vi "КАЛЬКУЛЯТОР.vi"() -> ()   [LabVIEW 2012]
uses:
  Control 1.ctl
panel:
  out "Boolean":bool
  in  ",":bool
  in  "+/-":bool
  in  "1/x":bool
  in  "CE":bool
  in  "C":bool
  in  "Backspace":bool
  in  "MS":bool
  in  "MR":bool
  in  "MC":bool
  in  "x^2":bool
  in  "sqrt":bool
  in  "/":bool
  in  "*":bool
  in  "-":bool
  in  "0":bool
  in  "9":bool
  in  "8":bool
  in  "7":bool
  in  "6":bool
  in  "5":bool
  in  "4":bool
  in  "3":bool
  out "екран":string
  in  "=":bool
  in  "+":bool
  in  "2":bool
  in  "1":bool
  in  "stop":bool
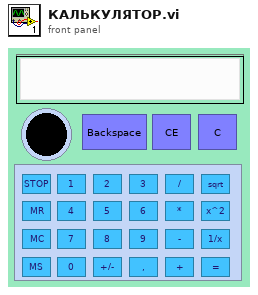
[diagram p1: front panel]
types:
  T1 = typedef "Control 1.ctl" = enum16{",", "+/-", "1/x", "Backspace", "CE", "C", "MC", "MR", "MS", "x^2", "sqrt", "поділити", "помножити", "відняти", "0", "9", "8", "7", "6", "5", "4", "3", "1", "2", "додати", "дорівнює", "стоп"}
  T2 = cluster{"екран":string, "чис ек":string, "буф":string, "Enum":T1, "MR":string, "MS":string}
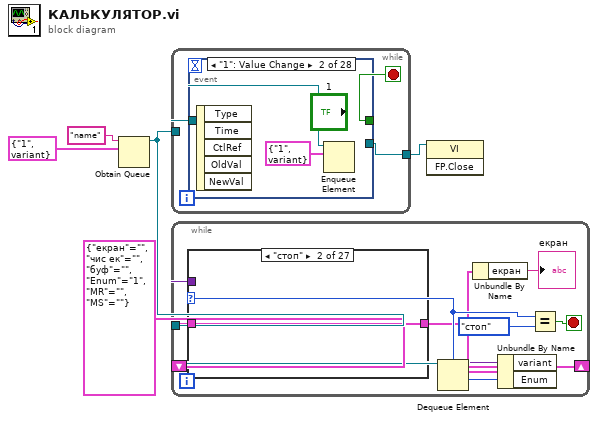
[diagram p0: block diagram]
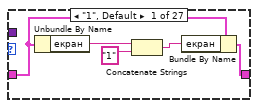
[diagram p2: hidden frame]
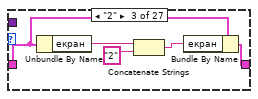
[diagram p3: hidden frame]
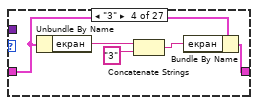
[diagram p4: hidden frame]
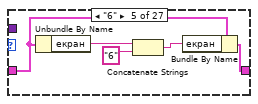
[diagram p5: hidden frame]
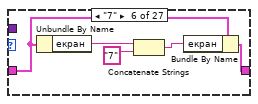
[diagram p6: hidden frame]
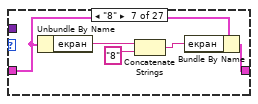
[diagram p7: hidden frame]
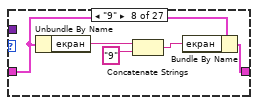
[diagram p8: hidden frame]
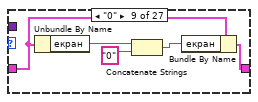
[diagram p9: hidden frame]
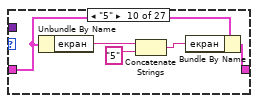
[diagram p10: hidden frame]
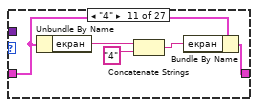
[diagram p11: hidden frame]
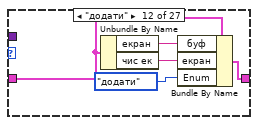
[diagram p12: hidden frame]
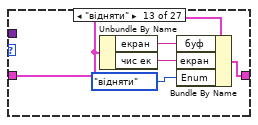
[diagram p13: hidden frame]
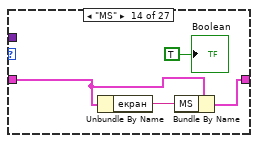
[diagram p14: hidden frame]
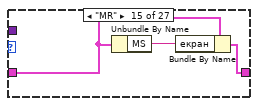
[diagram p15: hidden frame]
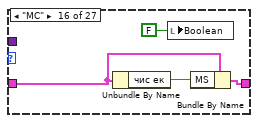
[diagram p16: hidden frame]
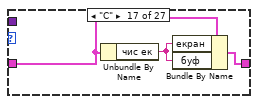
[diagram p17: hidden frame]
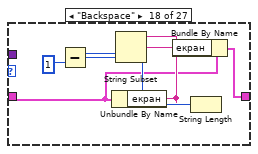
[diagram p18: hidden frame]
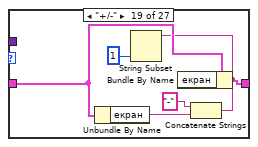
[diagram p19: hidden frame]
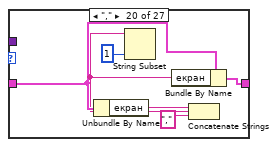
[diagram p20: hidden frame]
diagram:
  n1 = Obtain Queue(name (unnamed)="name", element data type=cluster{"Enum":T1, "variant":variant} {"Enum"=enum."1", "variant"=variant}) -> (queue out=w3:refnum<queue>)  [unwired: 3 in, 2 out]
  n2 = while {
    tunnel: w3 -> [w8]
    tunnel: [w6] -> w1
    stop <- w7 stop-if-true
    n3 = event shown="[1] \"1\": Value Change" {
      selector: _ -> [_ _ _ _ _ _ _ _ _ _ _ _ _ _ _ _ _ _ _ _ _ _ _ _ _ _ _ _]
      dyn-events: _ -> [_ _ _ _ _ _ _ _ _ _ _ _ _ _ _ _ _ _ _ _ _ _ _ _ _ _ _ _]
      timeout: _ -> [_ _ _ _ _ _ _ _ _ _ _ _ _ _ _ _ _ _ _ _ _ _ _ _ _ _ _ _]
      tunnel: w8 -> [w11 w14 w15 w17 w19 w21 w23 w25 w29 w43 w45 w47 w49 w52 w54 w56 w58 w60 w62 w64 w66 w68 w70 w72 w74 w76 w77 w80]
      tunnel: ["stop" _ _ _ _ _ _ _ w27 _ _ _ _ _ _ _ _ _ _ _ _ _ _ _ _ _ _ _] -> w7
      tunnel: [w10 _ _ _ _ _ _ _ w28 _ _ _ _ _ _ _ _ _ _ _ _ _ _ _ _ _ _ _] -> w6
      event "stop": Value Change {
        n4 = event-data() -> ()  [unwired: 1 in, 2 out]
        n5 = Enqueue Element(queue=w11, element=cluster{"Enum":T1, "variant":variant} {"Enum"=enum."стоп", "variant"=variant}) -> ()  [unwired: 2 in, 3 out]
        n6 = control-ref of="This VI"() -> (w10:refnum<vi>)
      }
      event "1": Value Change {
        n7 = event-data() -> ()  [unwired: 1 in, 5 out]
        n8 = Enqueue Element(queue=w14, element=cluster{"Enum":T1, "variant":variant} {"Enum"=enum."1", "variant"=variant}) -> ()  [unwired: 2 in, 3 out]
      }
      event "3": Value Change {
        n9 = event-data() -> ()  [unwired: 1 in, 5 out]
        n10 = Enqueue Element(queue=w15, element=cluster{"Enum":T1, "variant":variant} {"Enum"=enum."3", "variant"=variant}) -> ()  [unwired: 2 in, 3 out]
      }
      event "4": Value Change {
        n11 = event-data() -> ()  [unwired: 1 in, 5 out]
        n12 = Enqueue Element(queue=w17, element=cluster{"Enum":T1, "variant":variant} {"Enum"=enum."4", "variant"=variant}) -> ()  [unwired: 2 in, 3 out]
      }
      event "+/-": Value Change {
        n13 = event-data() -> ()  [unwired: 1 in, 5 out]
        n14 = Enqueue Element(queue=w19, element=cluster{"Enum":T1, "variant":variant} {"Enum"=enum."+/-", "variant"=variant}) -> ()  [unwired: 2 in, 3 out]
      }
      event ",": Value Change {
        n15 = event-data() -> ()  [unwired: 1 in, 5 out]
        n16 = Enqueue Element(queue=w21, element=cluster{"Enum":T1, "variant":variant} {"Enum"=enum.",", "variant"=variant}) -> ()  [unwired: 2 in, 3 out]
      }
      event "5": Value Change {
        n17 = event-data() -> ()  [unwired: 1 in, 5 out]
        n18 = Enqueue Element(queue=w23, element=cluster{"Enum":T1, "variant":variant} {"Enum"=enum."5", "variant"=variant}) -> ()  [unwired: 2 in, 3 out]
      }
      event "0": Value Change {
        n19 = event-data() -> ()  [unwired: 1 in, 5 out]
        n20 = Enqueue Element(queue=w25, element=cluster{"Enum":T1, "variant":variant} {"Enum"=enum."0", "variant"=variant}) -> ()  [unwired: 2 in, 3 out]
      }
      event Menu Selection (User) {
        n21 = event-data() -> ("ItemTag"=w30:string)  [unwired: 1 in, 5 out]
        n22 = case shown="\"False\", Default" w30 {
          tunnel: w29 -> [_ w31 w33 w35 w37 w41]
          tunnel: [_ _ _ _ _ w40] -> w28
          tunnel: [_ _ _ _ _ TRUE] -> w27
          frame "False", Default {
          }
          frame "відняти" {
            n23 = Enqueue Element(queue=w31, element=cluster{"Enum":T1, "variant":variant} {"Enum"=enum."відняти", "variant"=variant}) -> ()  [unwired: 2 in, 3 out]
          }
          frame "додати" {
            n24 = Enqueue Element(queue=w33, element=cluster{"Enum":T1, "variant":variant} {"Enum"=enum."додати", "variant"=variant}) -> ()  [unwired: 2 in, 3 out]
          }
          frame "помножити" {
            n25 = Enqueue Element(queue=w35, element=cluster{"Enum":T1, "variant":variant} {"Enum"=enum."помножити", "variant"=variant}) -> ()  [unwired: 2 in, 3 out]
          }
          frame "поділити" {
            n26 = Enqueue Element(queue=w37, element=cluster{"Enum":T1, "variant":variant} {"Enum"=enum."поділити", "variant"=variant}) -> ()  [unwired: 2 in, 3 out]
          }
          frame "стоп" {
            n27 = control-ref of="This VI"() -> (w40:refnum<vi>)
            n28 = Enqueue Element(queue=w41, element=cluster{"Enum":T1, "variant":variant} {"Enum"=enum."стоп", "variant"=variant}) -> ()  [unwired: 2 in, 3 out]
          }
        }
      }
      event "6": Value Change {
        n29 = event-data() -> ()  [unwired: 1 in, 5 out]
        n30 = Enqueue Element(queue=w43, element=cluster{"Enum":T1, "variant":variant} {"Enum"=enum."6", "variant"=variant}) -> ()  [unwired: 2 in, 3 out]
      }
      event "7": Value Change {
        n31 = event-data() -> ()  [unwired: 1 in, 5 out]
        n32 = Enqueue Element(queue=w45, element=cluster{"Enum":T1, "variant":variant} {"Enum"=enum."7", "variant"=variant}) -> ()  [unwired: 2 in, 3 out]
      }
      event "8": Value Change {
        n33 = event-data() -> ()  [unwired: 1 in, 5 out]
        n34 = Enqueue Element(queue=w47, element=cluster{"Enum":T1, "variant":variant} {"Enum"=enum."8", "variant"=variant}) -> ()  [unwired: 2 in, 3 out]
      }
      event "9": Value Change {
        n35 = event-data() -> ()  [unwired: 1 in, 5 out]
        n36 = Enqueue Element(queue=w49, element=cluster{"Enum":T1, "variant":variant} {"Enum"=enum."9", "variant"=variant}) -> ()  [unwired: 2 in, 3 out]
      }
      event "+": Value Change {
        n37 = event-data() -> ()  [unwired: 1 in, 5 out]
        n38 = Enqueue Element(queue=w52, element=cluster{"Enum":T1, "variant":variant} {"Enum"=enum."додати", "variant"=variant}) -> ()  [unwired: 2 in, 3 out]
      }
      event "-": Value Change {
        n39 = event-data() -> ()  [unwired: 1 in, 5 out]
        n40 = Enqueue Element(queue=w54, element=cluster{"Enum":T1, "variant":variant} {"Enum"=enum."відняти", "variant"=variant}) -> ()  [unwired: 2 in, 3 out]
      }
      event "*": Value Change {
        n41 = event-data() -> ()  [unwired: 1 in, 5 out]
        n42 = Enqueue Element(queue=w56, element=cluster{"Enum":T1, "variant":variant} {"Enum"=enum."помножити", "variant"=variant}) -> ()  [unwired: 2 in, 3 out]
      }
      event "/": Value Change {
        n43 = event-data() -> ()  [unwired: 1 in, 5 out]
        n44 = Enqueue Element(queue=w58, element=cluster{"Enum":T1, "variant":variant} {"Enum"=enum."поділити", "variant"=variant}) -> ()  [unwired: 2 in, 3 out]
      }
      event "sqrt": Value Change {
        n45 = event-data() -> ()  [unwired: 1 in, 5 out]
        n46 = Enqueue Element(queue=w60, element=cluster{"Enum":T1, "variant":variant} {"Enum"=enum."sqrt", "variant"=variant}) -> ()  [unwired: 2 in, 3 out]
      }
      event "x^2": Value Change {
        n47 = event-data() -> ()  [unwired: 1 in, 5 out]
        n48 = Enqueue Element(queue=w62, element=cluster{"Enum":T1, "variant":variant} {"Enum"=enum."x^2", "variant"=variant}) -> ()  [unwired: 2 in, 3 out]
      }
      event "MC": Value Change {
        n49 = event-data() -> ()  [unwired: 1 in, 5 out]
        n50 = Enqueue Element(queue=w64, element=cluster{"Enum":T1, "variant":variant} {"Enum"=enum."MC", "variant"=variant}) -> ()  [unwired: 2 in, 3 out]
      }
      event "MR": Value Change {
        n51 = event-data() -> ()  [unwired: 1 in, 5 out]
        n52 = Enqueue Element(queue=w66, element=cluster{"Enum":T1, "variant":variant} {"Enum"=enum."MR", "variant"=variant}) -> ()  [unwired: 2 in, 3 out]
      }
      event "MS": Value Change {
        n53 = event-data() -> ()  [unwired: 1 in, 5 out]
        n54 = Enqueue Element(queue=w68, element=cluster{"Enum":T1, "variant":variant} {"Enum"=enum."MS", "variant"=variant}) -> ()  [unwired: 2 in, 3 out]
      }
      event "Backspace": Value Change {
        n55 = event-data() -> ()  [unwired: 1 in, 5 out]
        n56 = Enqueue Element(queue=w70, element=cluster{"Enum":T1, "variant":variant} {"Enum"=enum."Backspace", "variant"=variant}) -> ()  [unwired: 2 in, 3 out]
      }
      event "1/x": Value Change {
        n57 = event-data() -> ()  [unwired: 1 in, 5 out]
        n58 = Enqueue Element(queue=w72, element=cluster{"Enum":T1, "variant":variant} {"Enum"=enum."1/x", "variant"=variant}) -> ()  [unwired: 2 in, 3 out]
      }
      event "C": Value Change {
        n59 = event-data() -> ()  [unwired: 1 in, 5 out]
        n60 = Enqueue Element(queue=w74, element=cluster{"Enum":T1, "variant":variant} {"Enum"=enum."C", "variant"=variant}) -> ()  [unwired: 2 in, 3 out]
      }
      event "CE": Value Change {
        n61 = event-data() -> ()  [unwired: 1 in, 5 out]
        n62 = Enqueue Element(queue=w76, element=cluster{"Enum":T1, "variant":variant} {"Enum"=enum."CE", "variant"=variant}) -> ()  [unwired: 2 in, 3 out]
      }
      event "=": Value Change {
        n63 = event-data() -> ()  [unwired: 1 in, 5 out]
        n64 = Enqueue Element(queue=w77, element=cluster{"Enum":T1, "variant":variant} {"Enum"=enum."дорівнює", "variant"=variant}) -> ()  [unwired: 2 in, 3 out]
      }
      event "2": Value Change {
        n65 = event-data() -> ()  [unwired: 1 in, 5 out]
        n66 = Enqueue Element(queue=w80, element=cluster{"Enum":T1, "variant":variant} {"Enum"=enum."2", "variant"=variant}) -> ()  [unwired: 2 in, 3 out]
      }
    }
  }
  n67 = while {
    tunnel: w3 -> [w89]
    shift-right: [w83] -> _
    shift-left: T2 {"екран"="", "чис ек"="", "буф"="", "Enum"=enum."1", "MR"="", "MS"=""} -> [w84]
    stop <- w87 stop-if-true
    n68 = Dequeue Element(queue=w89) -> (element=w88:cluster{"Enum":T1, "variant":variant})  [unwired: 2 in, 3 out]
    n69 = Unbundle By Name(w88) -> ("variant"=w81:variant, "Enum"=w85:T1)
    n70 = case shown="\"стоп\"" w85 {
      tunnel: w84 -> [w91 w95 w100 w102 w106 w112 w116 w122 w127 w131 w137 w145 w150 w154 w157 w161 w164 w166 w176 w182 w186 w191 w196 w202 w208 w214 w216]
      tunnel: [w90 w95 w99 w101 w107 w111 w117 w121 w126 w132 w136 w141 w146 w153 w156 w160 w163 w165 w177 w183 w185 w187 w192 w201 w207 w213 w215] -> w83
      tunnel: w81 -> [_ _ _ _ _ _ _ _ _ _ _ _ _ _ _ _ _ _ _ _ _ _ _ _ _ _ _]
      frame "1", Default {
        n71 = Unbundle By Name(w91) -> ("екран"=w94:string)
        n72 = Concatenate Strings(w94, "1" ("string")) -> (w92:string)
        n73 = Bundle By Name(cluster=w91, "екран"=w92) -> (w90:T2)
      }
      frame "стоп" {
      }
      frame "2" {
        n74 = Unbundle By Name(w100) -> ("екран"=w98:string)
        n75 = Concatenate Strings(w98, "2" ("string")) -> (w96:string)
        n76 = Bundle By Name(cluster=w100, "екран"=w96) -> (w99:T2)
      }
      frame "3" {
        n77 = Unbundle By Name(w102) -> ("екран"=w103:string)
        n78 = Concatenate Strings(w103, "3" ("string")) -> (w105:string)
        n79 = Bundle By Name(cluster=w102, "екран"=w105) -> (w101:T2)
      }
      frame "6" {
        n80 = Unbundle By Name(w106) -> ("екран"=w110:string)
        n81 = Concatenate Strings(w110, "6" ("string")) -> (w108:string)
        n82 = Bundle By Name(cluster=w106, "екран"=w108) -> (w107:T2)
      }
      frame "7" {
        n83 = Unbundle By Name(w112) -> ("екран"=w113:string)
        n84 = Concatenate Strings(w113, "7" ("string")) -> (w115:string)
        n85 = Bundle By Name(cluster=w112, "екран"=w115) -> (w111:T2)
      }
      frame "8" {
        n86 = Unbundle By Name(w116) -> ("екран"=w120:string)
        n87 = Concatenate Strings(w120, "8" ("string")) -> (w118:string)
        n88 = Bundle By Name(cluster=w116, "екран"=w118) -> (w117:T2)
      }
      frame "9" {
        n89 = Unbundle By Name(w122) -> ("екран"=w123:string)
        n90 = Concatenate Strings(w123, "9" ("string")) -> (w125:string)
        n91 = Bundle By Name(cluster=w122, "екран"=w125) -> (w121:T2)
      }
      frame "0" {
        n92 = Unbundle By Name(w127) -> ("екран"=w128:string)
        n93 = Concatenate Strings(w128, "0" ("string")) -> (w130:string)
        n94 = Bundle By Name(cluster=w127, "екран"=w130) -> (w126:T2)
      }
      frame "5" {
        n95 = Unbundle By Name(w131) -> ("екран"=w135:string)
        n96 = Concatenate Strings(w135, "5" ("string")) -> (w133:string)
        n97 = Bundle By Name(cluster=w131, "екран"=w133) -> (w132:T2)
      }
      frame "4" {
        n98 = Unbundle By Name(w137) -> ("екран"=w138:string)
        n99 = Concatenate Strings(w138, "4" ("string")) -> (w140:string)
        n100 = Bundle By Name(cluster=w137, "екран"=w140) -> (w136:T2)
      }
      frame "додати" {
        n101 = Unbundle By Name(w145) -> ("екран"=w143:string, "чис ек"=w144:string)
        n102 = Bundle By Name(cluster=w145, "буф"=w143, "екран"=w144, "Enum"=Control_1."додати") -> (w141:T2)
      }
      frame "відняти" {
        n103 = Unbundle By Name(w150) -> ("екран"=w149:string, "чис ек"=w148:string)
        n104 = Bundle By Name(cluster=w150, "буф"=w149, "екран"=w148, "Enum"=Control_1."відняти") -> (w146:T2)
      }
      frame "MS" {
        n105 = Unbundle By Name(w154) -> ("екран"=w152:string)
        n106 = Bundle By Name(cluster=w154, "MS"=w152) -> (w153:T2)
        "Boolean" <- TRUE
      }
      frame "MR" {
        n107 = Unbundle By Name(w157) -> ("MS"=w155:string)
        n108 = Bundle By Name(cluster=w157, "екран"=w155) -> (w156:T2)
      }
      frame "MC" {
        n109 = Unbundle By Name(w161) -> ("чис ек"=w159:string)
        n110 = local write "Boolean"(FALSE) -> ()
        n111 = Bundle By Name(cluster=w161, "MS"=w159) -> (w160:T2)
      }
      frame "C" {
        n112 = Unbundle By Name(w164) -> ("чис ек"=w162:string)
        n113 = Bundle By Name(cluster=w164, "екран"=w162, "буф"=w162) -> (w163:T2)
      }
      frame "Backspace" {
        n114 = Unbundle By Name(w166) -> ("екран"=w168:string)
        n115 = String Length(string=w168) -> (length=w171:i32)
        n116 = Subtract(x=w171, y=1) -> (x-y=w169:i32)
        n117 = String Subset(string=w168, length (rest)=w169) -> (substring=w167:string)  [unwired: 1 in]
        n118 = Bundle By Name(cluster=w166, "екран"=w167) -> (w165:T2)
      }
      frame "+/-" {
        n119 = Unbundle By Name(w176) -> ("екран"=w174:string)
        n120 = Concatenate Strings("-" ("string"), w174) -> (w173:string)
        n121 = String Subset(string=w173, length (rest)=1 ("length (rest)")) -> ()  [unwired: 1 in, 1 out]
        n122 = Bundle By Name(cluster=w176, "екран"=w173) -> (w177:T2)
      }
      frame "," {
        n123 = Unbundle By Name(w182) -> ("екран"=w179:string)
        n124 = Concatenate Strings(w179, "," ("string")) -> (w181:string)
        n125 = String Subset(string=w181, length (rest)=1 ("length (rest)")) -> ()  [unwired: 1 in, 1 out]
        n126 = Bundle By Name(cluster=w182, "екран"=w181) -> (w183:T2)
      }
      frame "CE" {
        n127 = Unbundle By Name(w186) -> ("чис ек"=w184:string)
        n128 = Bundle By Name(cluster=w186, "екран"=w184) -> (w185:T2)
      }
      frame "помножити" {
        n129 = Unbundle By Name(w191) -> ("екран"=w190:string, "чис ек"=w189:string)
        n130 = Bundle By Name(cluster=w191, "буф"=w190, "екран"=w189, "Enum"=Control_1."помножити") -> (w187:T2)
      }
      frame "поділити" {
        n131 = Unbundle By Name(w196) -> ("екран"=w195:string, "чис ек"=w194:string)
        n132 = Bundle By Name(cluster=w196, "буф"=w195, "екран"=w194, "Enum"=Control_1."поділити") -> (w192:T2)
      }
      frame "sqrt" {
        n133 = Unbundle By Name(w202) -> ("екран"=w200:string)
        n134 = Scan From String(input string=w200) -> (output 1=w198:dbl)  [unwired: 4 in, 3 out]
        n135 = Square Root(x=w198) -> (sqrt(x)=w197:dbl)
        n136 = Format Into String(w197) -> (resulting string=w199:string)  [unwired: 3 in, 1 out]
        n137 = Bundle By Name(cluster=w202, "екран"=w199) -> (w201:T2)
      }
      frame "x^2" {
        n138 = Unbundle By Name(w208) -> ("екран"=w206:string)
        n139 = Scan From String(input string=w206) -> (output 1=w204:dbl)  [unwired: 4 in, 3 out]
        n140 = Square(x=w204) -> (x^2=w203:dbl)
        n141 = Format Into String(w203) -> (resulting string=w205:string)  [unwired: 3 in, 1 out]
        n142 = Bundle By Name(cluster=w208, "екран"=w205) -> (w207:T2)
      }
      frame "1/x" {
        n143 = Unbundle By Name(w214) -> ("екран"=w212:string)
        n144 = Scan From String(input string=w212) -> (output 1=w210:dbl)  [unwired: 4 in, 3 out]
        n145 = Reciprocal(x=w210) -> (1/x=w209:dbl)
        n146 = Format Into String(w209) -> (resulting string=w211:string)  [unwired: 3 in, 1 out]
        n147 = Bundle By Name(cluster=w214, "екран"=w211) -> (w213:T2)
      }
      frame "дорівнює" {
        n148 = Unbundle By Name(w216) -> ("екран"=w223:string, "буф"=w222:string, "Enum"=w221:T1)
        n149 = Scan From String(input string=w223) -> (output 1=w219:dbl)  [unwired: 4 in, 3 out]
        n150 = Scan From String(input string=w222) -> (output 1=w220:dbl)  [unwired: 4 in, 3 out]
        n151 = case shown="\"поділити\"" w221 {
          tunnel: w220 -> [_ w227 w228 w233 w234]
          tunnel: w219 -> [w224 w226 w229 w232 w235]
          tunnel: [w224 w225 w230 w231 w236] -> w218
          frame "дорівнює", Default {
          }
          frame "додати" {
            n152 = Add(x=w226, y=w227) -> (x+y=w225:dbl)
          }
          frame "відняти" {
            n153 = Subtract(x=w228, y=w229) -> (x-y=w230:dbl)
          }
          frame "помножити" {
            n154 = Multiply(x=w232, y=w233) -> (x*y=w231:dbl)
          }
          frame "поділити" {
            n155 = Divide(x=w234, y=w235) -> (x/y=w236:dbl)
          }
        }
        n156 = Format Into String(w218) -> (resulting string=w217:string)  [unwired: 3 in, 1 out]
        n157 = Bundle By Name(cluster=w216, "екран"=w217) -> (w215:T2)
      }
    }
    n158 = Unbundle By Name(w83) -> ("екран"=→"екран":string)
    n159 = Equal?(x=w85, y=Control_1."стоп" ("Enum")) -> (x = y?=w87:bool)
  }
  n160 = invoke class="VI" method="FP.Close"(reference=w1) -> ()  [unwired: 2 in, 3 out]
